vi "to string.vi"(8 "error in":errorcluster, 11 "byte":u8[](array[numeric]) format="%b") -> (0 "error out":errorcluster, 3 "String":string)   [LabVIEW 2020, in "wamplv.lvlib" / "MessagePack.lvclass"]
uses:
  MessagePack.lvclass
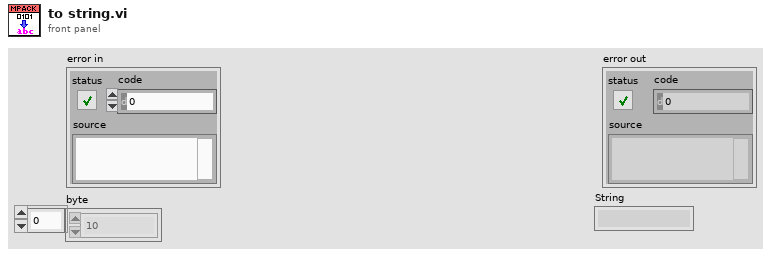
[diagram p1: front panel]
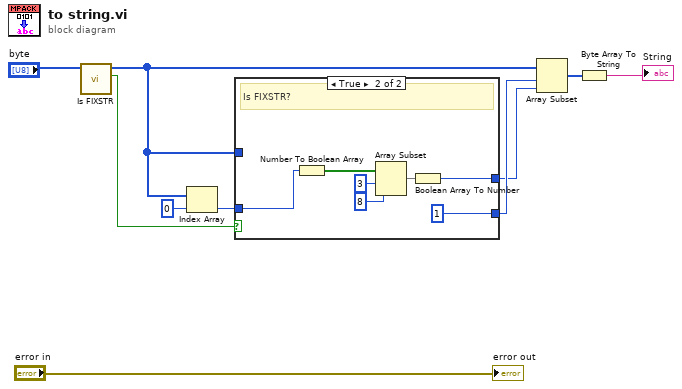
[diagram p0: block diagram]
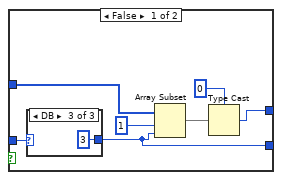
[diagram p2: hidden frame]
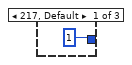
[diagram p3: hidden frame]
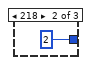
[diagram p4: hidden frame]
diagram:
  n1 = call "Is FIXSTR.vi"("bytes"="byte") -> ("Is FIXSTR?"=w9:bool, "bytes"=w5:u8[])  [unwired: 9 in]
  n2 = Index Array(array=w5, index=0) -> (element=w6:u8)
  n3 = case shown="True" w9 {
    tunnel: [w12 w24] -> w3
    tunnel: w6 -> [w17 w23]
    tunnel: [w11 u32 1] -> w4
    tunnel: w5 -> [w16 _]
    frame False {
      n4 = case shown="DB" w17 {
        tunnel: [1 2 3] -> w11
        frame 217, Default {
        }
        frame 218 {
        }
        frame 219 {
        }
      }
      n5 = Array Subset(array=w16, index=1, length=w11) -> (w14:u8[])
      n6 = Type Cast(type=u32 0, x=w14) -> (*(type *) &x=w12:u32)
    }
    frame True {
      # "Is FIXSTR?"
      n7 = Number To Boolean Array(number=w23) -> (Boolean array=w22:bool[])
      n8 = Array Subset(array=w22, index=3, length=8) -> (w25:bool[])
      n9 = Boolean Array To Number(Boolean array=w25) -> (number=w24:u32)
    }
  }
  n10 = Array Subset(array=w5, index=w4, length=w3) -> (w2:u8[])
  n11 = Byte Array To String(unsigned byte array=w2) -> (string=→"String":string)
  "error out" <- "error in"
